vi "RDUW_2.0.vi"() -> ()   [LabVIEW 2010]
panel:
  in  "Reset":bool
  out "Previous Write time (sec)":dbl
  in  "Start writing":bool
  out "Rubbish variable":bool
  out "XY Graph":cluster{"Y":dbl[], "Y":dbl[]}[](graph)
  in  "Monitor Motor Position":bool=TRUE
  out "Program runtime (s)":dbl format="%.1f"
  in  "Go Origin":bool
  in  "Emergency STOP !!":bool caption="Emergency Button"
  out "Output Array":dbl[][](array[numeric])
  in  "Command":string
  out "Loop count":i32
  out "y":i32
  out "x":i32
  out "x-disp":i32[](array[numeric])
  out "y-disp":i32[](array[numeric])
  in  "Laser GPIB":u8=10
  in  "Motor GPIB":u8=6
  # "1) LINE<space>[Displacement]<space>[Speed]<space>[Current]<space>[t(on)]<space>[t(off)]"
  # "2) JUMP<space>[Displacement]<space>[Speed]"
  # "3) ARC<space>[Type]<space>[Radius]<space>[Current]<space>[t(on)]<space>[t(off)]"
  # "4) LINE1<space>[Displacement]<space>[Speed]<space>[Current]<space>[t_before]<space>[t_enable]<space>[Frequency]<space>[DTY]<space>[HIL]<space>[LOL]"
  # "5) LINE2<space>[Displacement]<space>[Speed]<space>[Current]<space>[t_before]<space>[frequency]<space>[Amplitude]<space>[t_enable]"
  # "6) WAIT<space>[time_ms]"
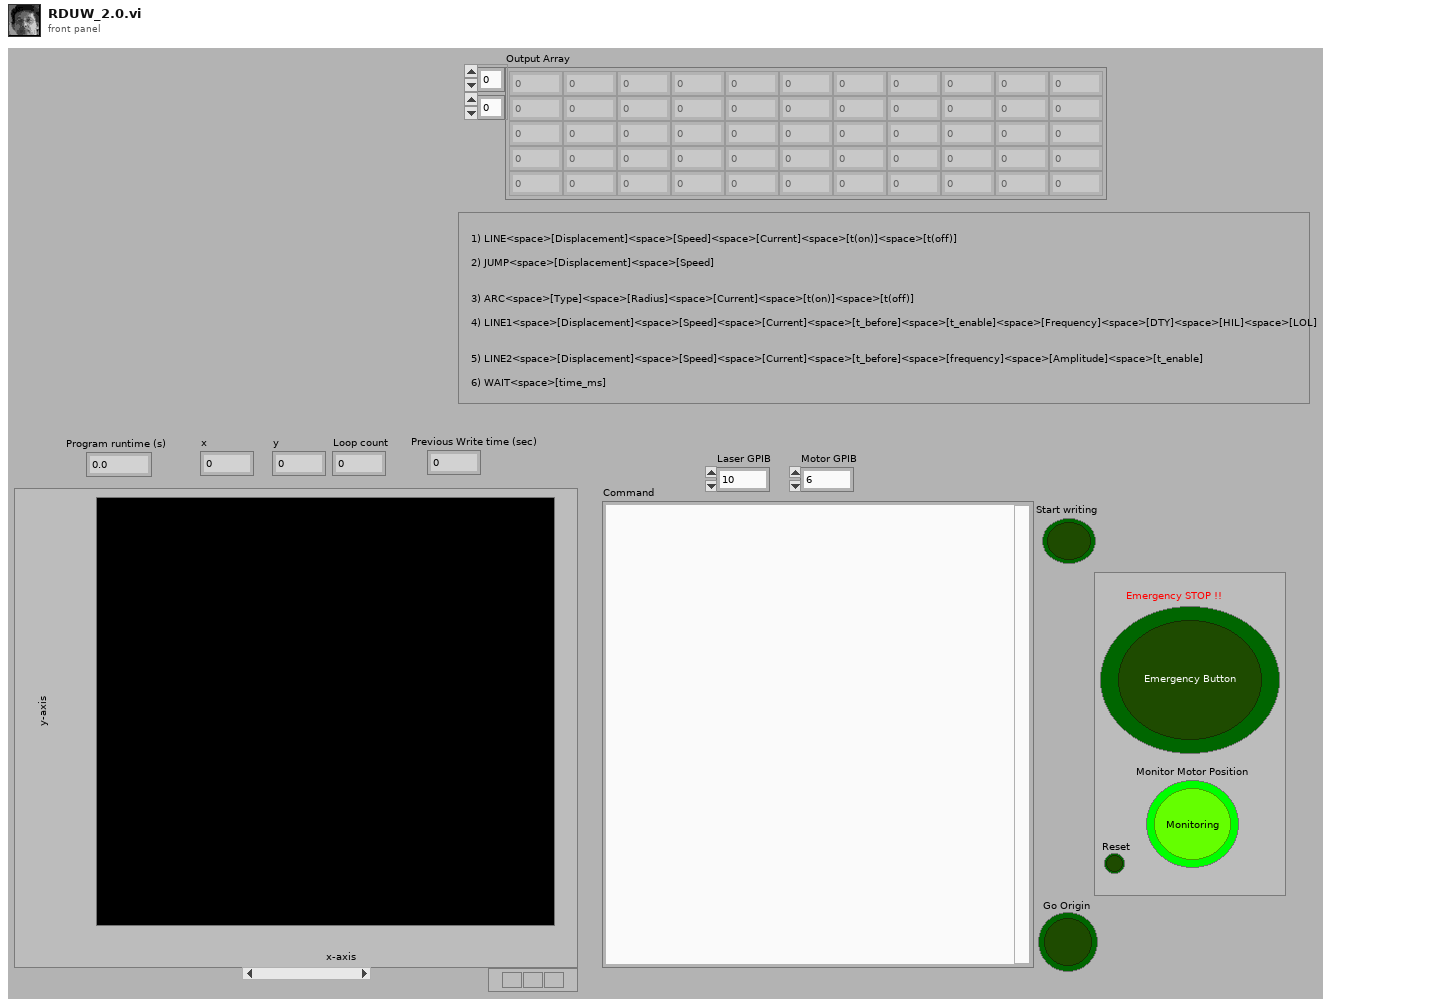
[diagram p1: front panel]
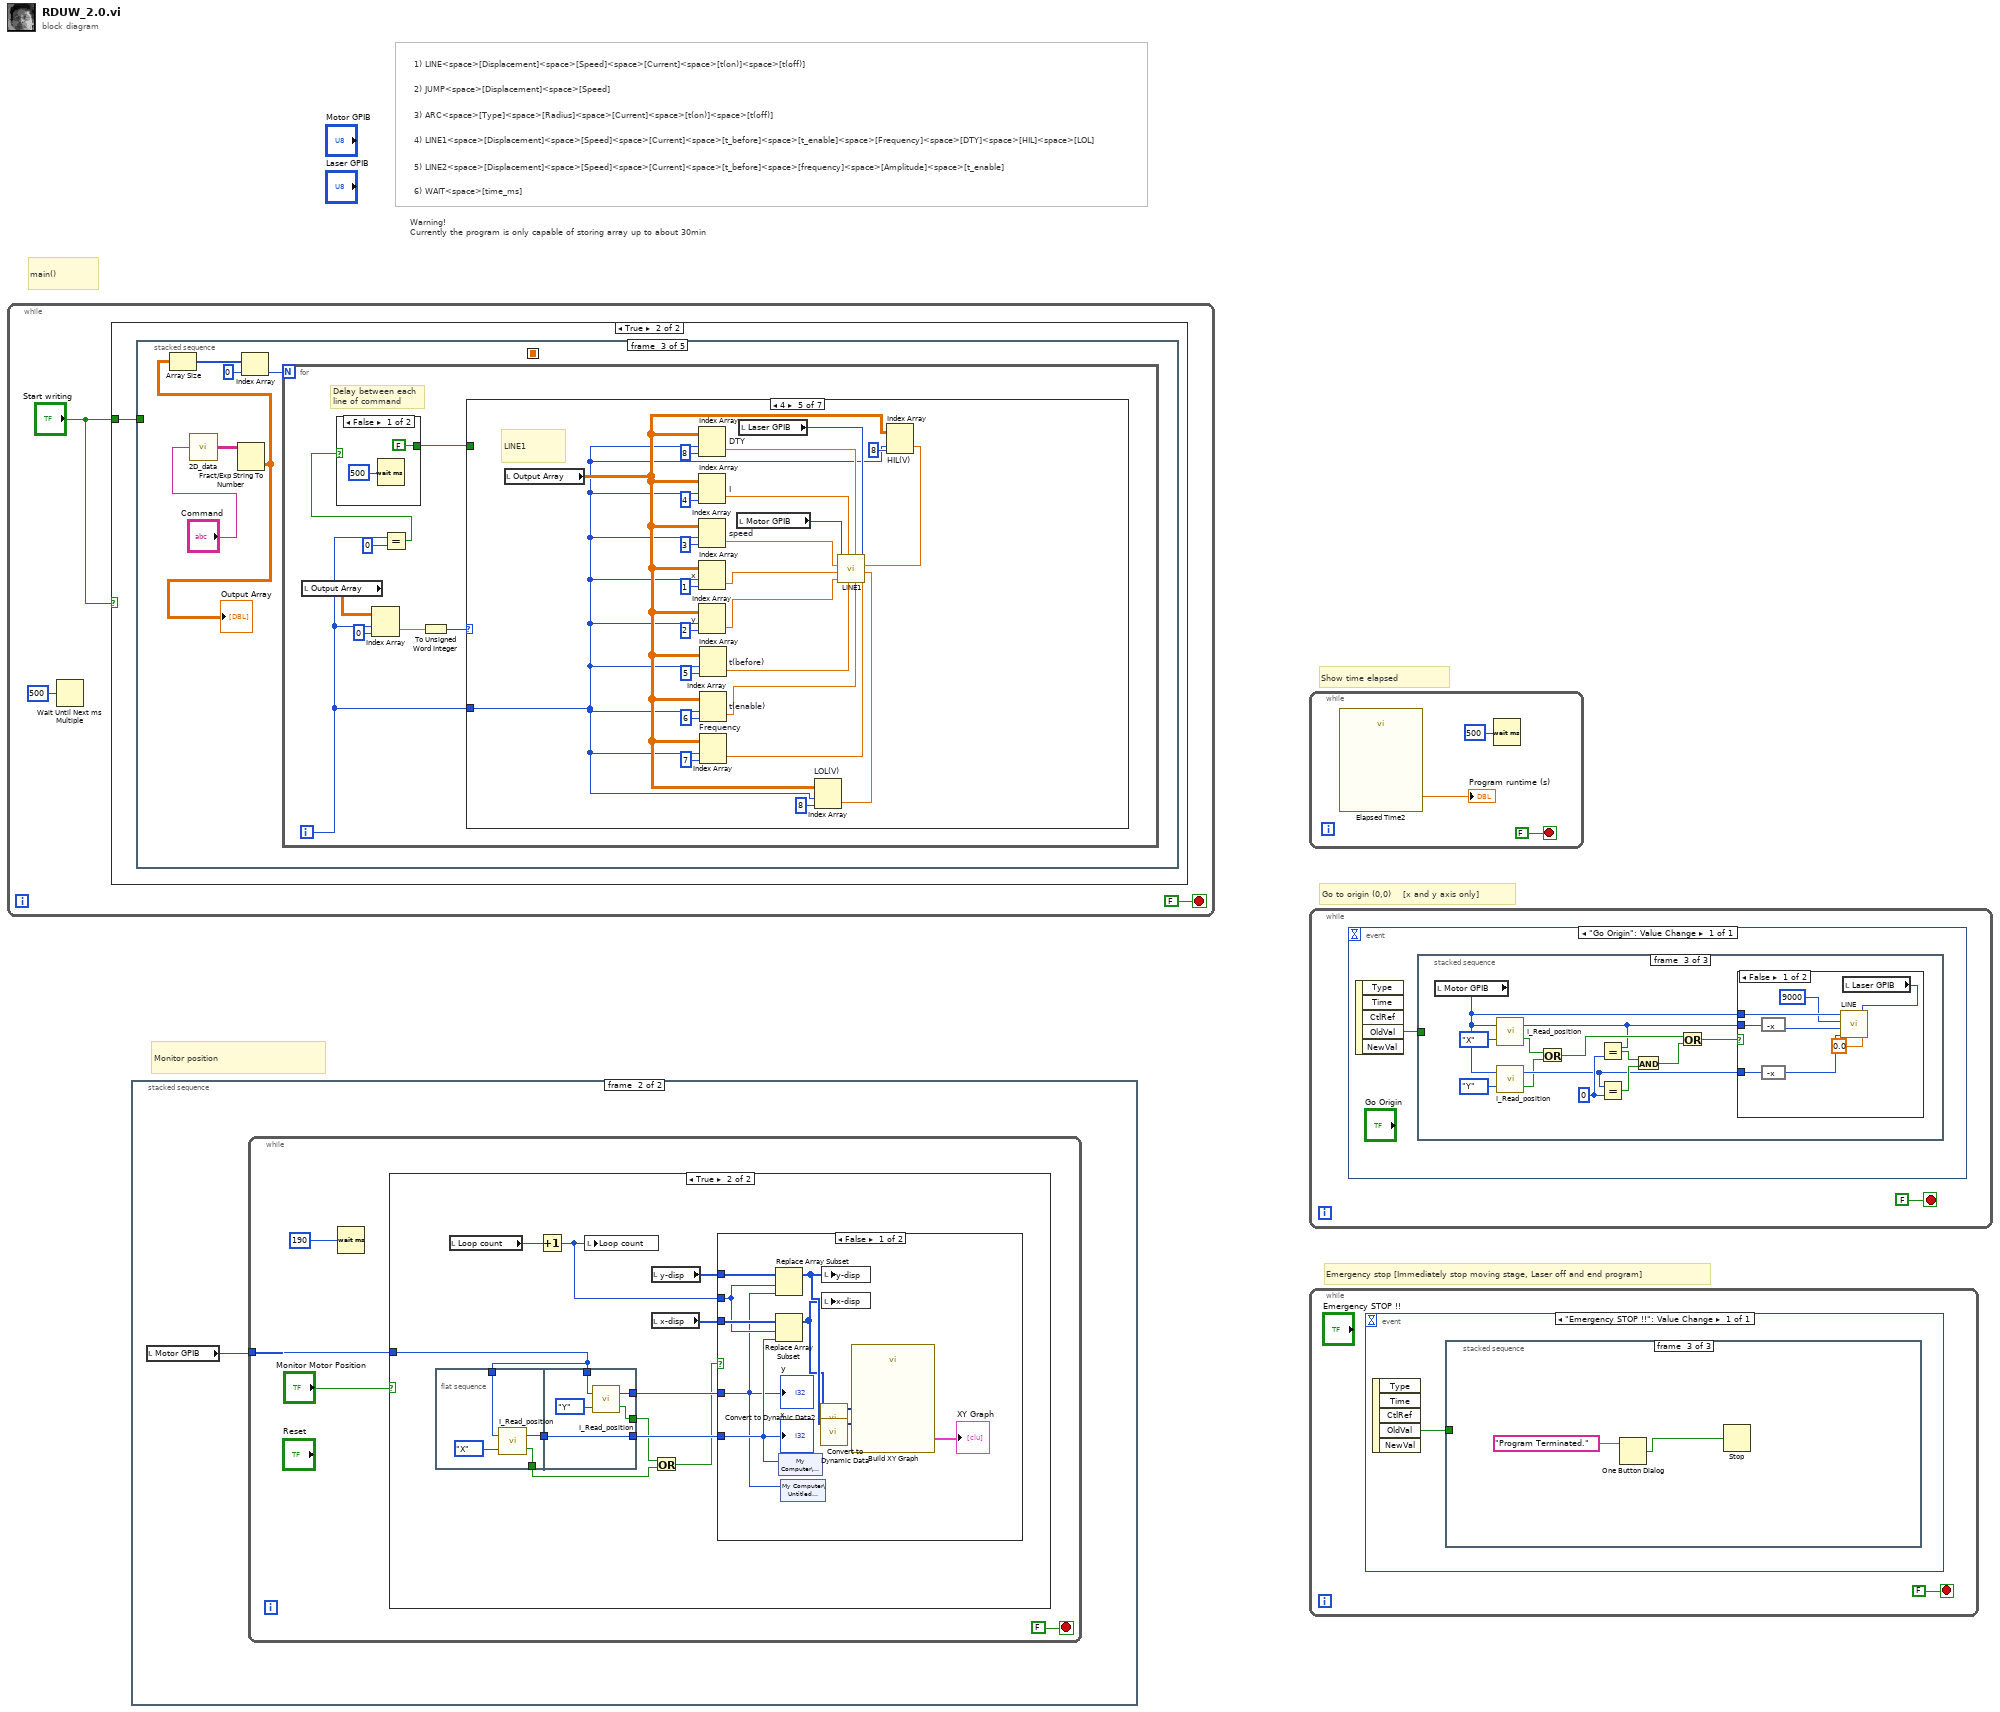
[diagram p0: block diagram]
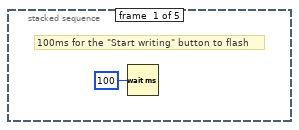
[diagram p3: hidden frame]
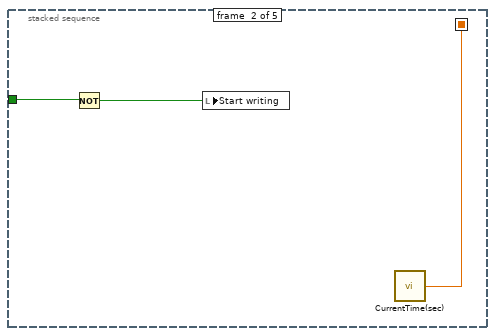
[diagram p4: hidden frame]
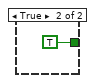
[diagram p5: hidden frame]
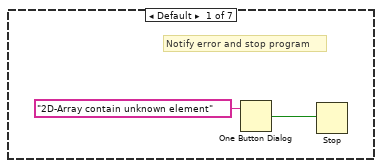
[diagram p6: hidden frame]
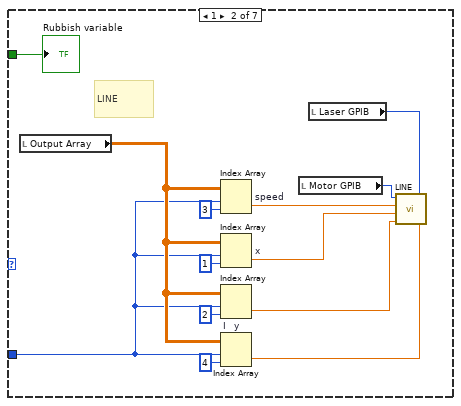
[diagram p7: hidden frame]
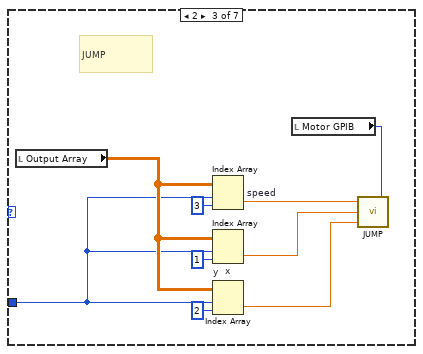
[diagram p8: hidden frame]
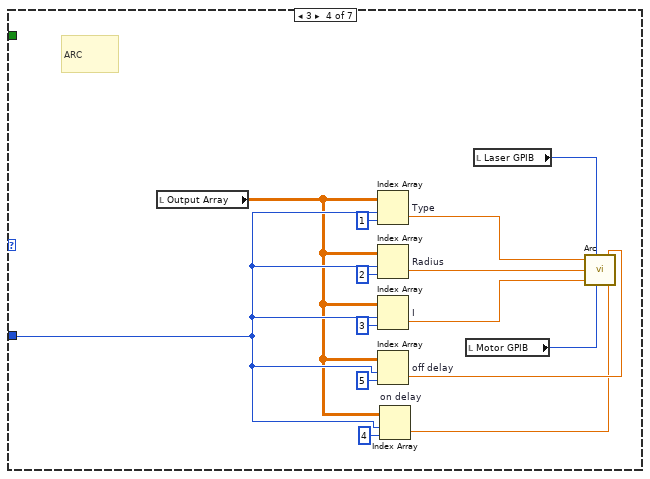
[diagram p9: hidden frame]
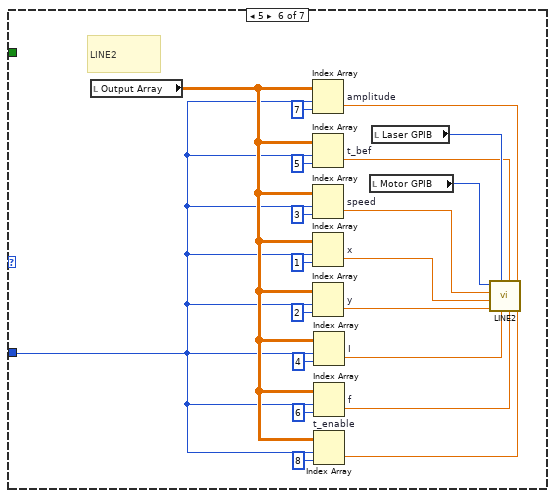
[diagram p10: hidden frame]
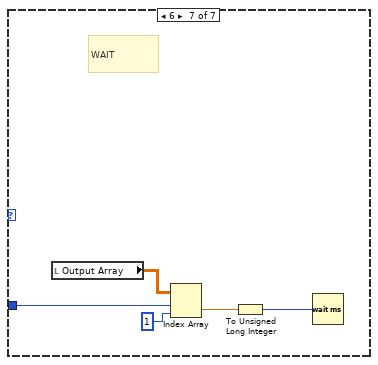
[diagram p11: hidden frame]
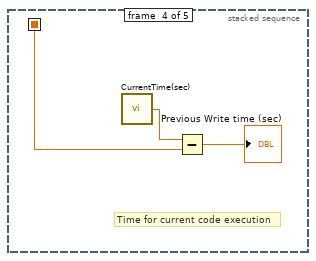
[diagram p12: hidden frame]
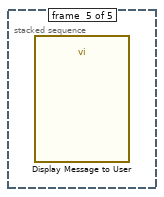
[diagram p13: hidden frame]
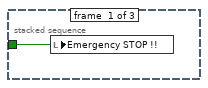
[diagram p14: hidden frame]
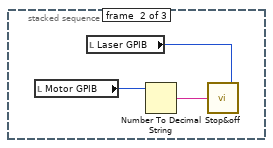
[diagram p15: hidden frame]
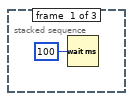
[diagram p16: hidden frame]
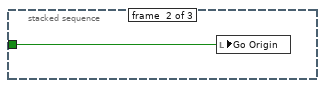
[diagram p17: hidden frame]
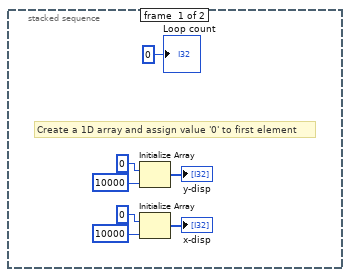
[diagram p19: hidden frame]
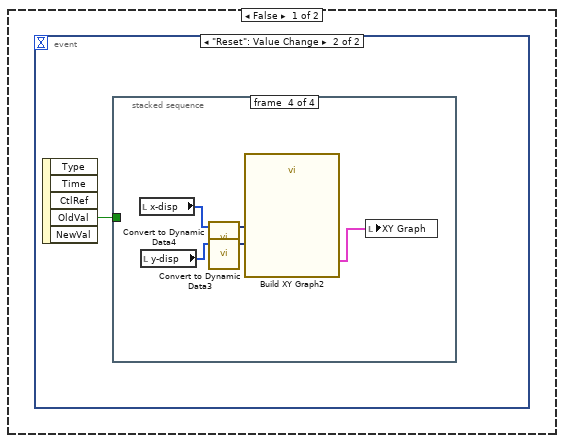
[diagram p20: hidden frame]
diagram:
  # "Warning!\nCurrently the program is only capable of storing array up to about 30min"
  # "main()"
  # "Emergency stop [Immediately stop moving stage, Laser off and end program]"
  # "Go to origin (0,0)    [x and y axis only]"
  # "Show time elapsed"
  # "6) WAIT<space>[time_ms]"
  # "5) LINE2<space>[Displacement]<space>[Speed]<space>[Current]<space>[t_before]<space>[frequency]<space>[Amplitude]<space>[t_enable]"
  # "Monitor position"
  # "4) LINE1<space>[Displacement]<space>[Speed]<space>[Current]<space>[t_before]<space>[t_enable]<space>[Frequency]<space>[DTY]<space>[HIL]<space>[LOL]"
  # "3) ARC<space>[Type]<space>[Radius]<space>[Current]<space>[t(on)]<space>[t(off)]"
  # "2) JUMP<space>[Displacement]<space>[Speed]"
  # "1) LINE<space>[Displacement]<space>[Speed]<space>[Current]<space>[t(on)]<space>[t(off)]"
  n1 = while {
    stop <- FALSE stop-if-true
    n2 = Wait Until Next ms Multiple(millisecond multiple=u32 500) -> ()  [unwired: 1 out]
    n3 = case shown="True" "Start writing" {
      tunnel: "Start writing" -> [_ w4]
      frame False {
      }
      frame True {
        n4 = stacked-sequence {
          seq-local: [_ w8 _ _ _] -> [_ _ _ w114 _]
          tunnel: w4 -> [_ w7 _ _ _]
          frame #0 {
            # "100ms for the \"Start writing\" button to flash"
            n5 = Wait (ms)(milliseconds to wait=u32 100) -> ()  [unwired: 1 out]
          }
          frame #1 {
            n6 = Not(x=w7) -> (.not. x?=w6:bool)
            n7 = local write "Start writing"(w6) -> ()
            n8 = call "CurrentTime(sec).vi"() -> ("CurrentTime(sec)"=w8:dbl)  [unwired: 1 in]
          }
          frame #2 {
            n9 = call "2D_data.vi"("String"="Command") -> ("output array"=w10:string[][])
            n10 = Fract/Exp String To Number(string=w10) -> (number=w9:dbl[][])  [unwired: 3 in, 1 out]
            "Output Array" <- w9
            n11 = Array Size(array=w9) -> (size(s)=w13:i32[])
            n12 = Index Array(array=w13, index=0) -> (element=w14:i32)
            n13 = for {
              N: w14 -> [_]
              i -> [w18]
              # "Delay between each\nline of command"
              n14 = local read "Output Array"() -> (w19:dbl[][])
              n15 = Index Array(array=w19, index (row)=w18, index (col)=0 ("disabled index (col)")) -> (element=w20:dbl)
              n16 = Equal?(x=w18, y=0) -> (x = y?=w16:bool)
              n17 = case shown="False" w16 {
                tunnel: [FALSE TRUE] -> w15
                frame False {
                  n18 = Wait (ms)(milliseconds to wait=u32 500) -> ()  [unwired: 1 out]
                }
                frame True {
                }
              }
              n19 = To Unsigned Word Integer(number=w20) -> (unsigned 16bit integer=w21:u16)
              n20 = case shown="4" w21 {
                tunnel: w18 -> [_ w28 w44 w63 w64 w88 w111]
                tunnel: w15 -> [_ w30 _ _ _ _ _]
                frame Default {
                  # "Notify error and stop program"
                  n21 = One Button Dialog(message="2D-Array contain unknown element") -> (true=w26:bool)  [unwired: 1 in]
                  n22 = Stop(stop? (T)=w26) -> ()
                }
                frame 1 {
                  # "LINE"
                  n23 = local read "Output Array"() -> (w29:dbl[][])
                  n24 = Index Array "speed"(array=w29, index (row)=w28, index (col)=3 ("disabled index (col)")) -> (element=w31:dbl)
                  n25 = Index Array "x"(array=w29, index (row)=w28, index (col)=1 ("disabled index (col)")) -> (element=w33:dbl)
                  n26 = Index Array "y"(array=w29, index (row)=w28, index (col)=2 ("disabled index (col)")) -> (element=w32:dbl)
                  n27 = Index Array "I"(array=w29, index (row)=w28, index (col)=4 ("disabled index (col)")) -> (element=w37:dbl)
                  n28 = local read "Motor GPIB"() -> (w39:u8)
                  n29 = local read "Laser GPIB"() -> (w40:u8)
                  n30 = call "LINE.vi"("Current (mA)"=w37, "Laser GPIB"=w40, "y-dist"=w32, "x-dist"=w33, "speed"=w31, "Motor GPIB"=w39) -> ()  [unwired: 2 in]
                  "Rubbish variable" <- w30
                }
                frame 2 {
                  # "JUMP"
                  n31 = local read "Output Array"() -> (w45:dbl[][])
                  n32 = Index Array "speed"(array=w45, index (row)=w44, index (col)=3 ("disabled index (col)")) -> (element=w43:dbl)
                  n33 = Index Array "x"(array=w45, index (row)=w44, index (col)=1 ("disabled index (col)")) -> (element=w42:dbl)
                  n34 = Index Array "y"(array=w45, index (row)=w44, index (col)=2 ("disabled index (col)")) -> (element=w41:dbl)
                  n35 = local read "Motor GPIB"() -> (w49:u8)
                  n36 = call "JUMP.vi"("Motor GPIB"=w49, "y-dist"=w41, "x-dist"=w42, "speed"=w43) -> ()
                }
                frame 3 {
                  # "ARC"
                  n37 = local read "Output Array"() -> (w52:dbl[][])
                  n38 = Index Array "Type"(array=w52, index (row)=w63, index (col)=1 ("disabled index (col)")) -> (element=w58:dbl)
                  n39 = Index Array "Radius"(array=w52, index (row)=w63, index (col)=2 ("disabled index (col)")) -> (element=w57:dbl)
                  n40 = Index Array "I"(array=w52, index (row)=w63, index (col)=3 ("disabled index (col)")) -> (element=w59:dbl)
                  n41 = Index Array "off delay"(array=w52, index (row)=w63, index (col)=5 ("disabled index (col)")) -> (element=w51:dbl)
                  n42 = Index Array "on delay"(array=w52, index (row)=w63, index (col)=4 ("disabled index (col)")) -> (element=w50:dbl)
                  n43 = local read "Motor GPIB"() -> (w55:u8)
                  n44 = local read "Laser GPIB"() -> (w56:u8)
                  n45 = call "Arc.vi"("Type"=w58, "Laser GPIB"=w56, "Radius"=w57, "Current (mA)"=w59, "Motor GPIB"=w55, "off delay"=w51, "on delay"=w50) -> ()
                }
                frame 4 {
                  # "LINE1"
                  n46 = local read "Output Array"() -> (w65:dbl[][])
                  n47 = Index Array "DTY"(array=w65, index (row)=w64, index (col)=8 ("disabled index (col)")) -> (element=w78:dbl)
                  n48 = Index Array "I"(array=w65, index (row)=w64, index (col)=4 ("disabled index (col)")) -> (element=w77:dbl)
                  n49 = Index Array "speed"(array=w65, index (row)=w64, index (col)=3 ("disabled index (col)")) -> (element=w76:dbl)
                  n50 = Index Array "x"(array=w65, index (row)=w64, index (col)=1 ("disabled index (col)")) -> (element=w75:dbl)
                  n51 = Index Array "y"(array=w65, index (row)=w64, index (col)=2 ("disabled index (col)")) -> (element=w74:dbl)
                  n52 = Index Array "t(before)"(array=w65, index (row)=w64, index (col)=5 ("disabled index (col)")) -> (element=w73:dbl)
                  n53 = Index Array "t(enable)"(array=w65, index (row)=w64, index (col)=6 ("disabled index (col)")) -> (element=w72:dbl)
                  n54 = Index Array "Frequency"(array=w65, index (row)=w64, index (col)=7 ("disabled index (col)")) -> (element=w71:dbl)
                  n55 = local read "Motor GPIB"() -> (w70:u8)
                  n56 = local read "Laser GPIB"() -> (w79:u8)
                  n57 = Index Array "LOL(V)"(array=w65, index (row)=w64, index (col)=8 ("disabled index (col)")) -> (element=w66:dbl)
                  n58 = Index Array "HIL(V)"(array=w65, index (row)=w64, index (col)=8 ("disabled index (col)")) -> (element=w67:dbl)
                  n59 = call "LINE1.vi"("Frequency(Hz)"=w71, "LOL(V)"=w66, "HIL(V)"=w67, "Laser GPIB"=w79, "Enable time(ms)"=w72, "DTY"=w78, "t_before(ms)"=w73, "Current (mA)"=w77, "y-dist"=w74, "x-dist"=w75, "speed"=w76, "Motor GPIB"=w70) -> ()
                }
                frame 5 {
                  # "LINE2"
                  n60 = local read "Output Array"() -> (w99:dbl[][])
                  n61 = Index Array "amplitude"(array=w99, index (row)=w88, index (col)=7 ("disabled index (col)")) -> (element=w90:dbl)
                  n62 = Index Array "t_bef"(array=w99, index (row)=w88, index (col)=5 ("disabled index (col)")) -> (element=w91:dbl)
                  n63 = Index Array "speed"(array=w99, index (row)=w88, index (col)=3 ("disabled index (col)")) -> (element=w95:dbl)
                  n64 = Index Array "x"(array=w99, index (row)=w88, index (col)=1 ("disabled index (col)")) -> (element=w96:dbl)
                  n65 = Index Array "y"(array=w99, index (row)=w88, index (col)=2 ("disabled index (col)")) -> (element=w94:dbl)
                  n66 = Index Array "I"(array=w99, index (row)=w88, index (col)=4 ("disabled index (col)")) -> (element=w93:dbl)
                  n67 = Index Array "f"(array=w99, index (row)=w88, index (col)=6 ("disabled index (col)")) -> (element=w92:dbl)
                  n68 = Index Array "t_enable"(array=w99, index (row)=w88, index (col)=8 ("disabled index (col)")) -> (element=w89:dbl)
                  n69 = local read "Motor GPIB"() -> (w98:u8)
                  n70 = local read "Laser GPIB"() -> (w97:u8)
                  n71 = call "LINE2.vi"("Enable time(ms)"=w89, "Amplitude(mV)"=w90, "Frequency(Hz)"=w92, "t_before(ms)"=w91, "Current (mA)"=w93, "Laser GPIB"=w97, "y-dist"=w94, "x-dist"=w96, "speed"=w95, "Motor GPIB"=w98) -> ()  [unwired: 2 in]
                }
                frame 6 {
                  # "WAIT"
                  n72 = local read "Output Array"() -> (w110:dbl[][])
                  n73 = Index Array "Index array"(array=w110, index (row)=w111, index (col)=1 ("disabled index (col)")) -> (element=w109:dbl)
                  n74 = To Unsigned Long Integer(number=w109) -> (unsigned 32bit integer=w108:u32)
                  n75 = Wait (ms)(milliseconds to wait=w108) -> ()  [unwired: 1 out]
                }
              }
            }
          }
          frame #3 {
            # "Time for current code execution"
            n76 = call "CurrentTime(sec).vi"() -> ("CurrentTime(sec)"=w115:dbl)  [unwired: 1 in]
            n77 = Subtract(x=w115, y=w114) -> (x-y=→"Previous Write time (sec)":dbl)
          }
          frame #4 {
            n78 = call "Display Message to User"() -> ()  [unwired: 10 in, 2 out]
          }
        }
      }
    }
  }
  n79 = stacked-sequence {
    frame #0 {
      # "Create a 1D array and assign value '0' to first element"
      n80 = Initialize Array(0 ("element"), 10000 ("dimension size")) -> (→"y-disp":i32[])
      n81 = Initialize Array(0 ("element"), 10000 ("element")) -> (→"x-disp":i32[])
      "Loop count" <- 0 ("Loop count")
    }
    frame #1 {
      n82 = local read "Motor GPIB"() -> (w123:u8)
      n83 = while {
        tunnel: w123 -> [w127]
        stop <- FALSE stop-if-true
        n84 = Wait (ms)(milliseconds to wait=u32 190 ("millisecond multiple")) -> ()  [unwired: 1 out]
        n85 = case shown="True" "Monitor Motor Position" {
          tunnel: w127 -> [_ w152]
          frame False {
            n86 = event shown="[1] \"Reset\": Value Change" {
              selector: _ -> [_ _]
              dyn-events: _ -> [_ _]
              timeout: _ -> [_ _]
              event "Monitor Motor Position": Value Change {
                n87 = event-data() -> ()  [unwired: 1 in, 5 out]
              }
              event "Reset": Value Change {
                n88 = event-data() -> ("OldVal"=w128:bool)  [unwired: 1 in, 4 out]
                n89 = stacked-sequence {
                  tunnel: w128 -> [_ w130 _ _]
                  frame #0 {
                    n90 = Wait (ms)(milliseconds to wait=u32 100) -> ()  [unwired: 1 out]
                  }
                  frame #1 {
                    n91 = local write "Reset"(w130) -> ()
                  }
                  frame #2 {
                    n92 = Initialize Array(0 ("element"), 10000 ("dimension size")) -> (w131:i32[])
                    n93 = Initialize Array(0 ("element"), 10000 ("element")) -> (w132:i32[])
                    n94 = local write "x-disp"(w131) -> ()
                    n95 = local write "y-disp"(w132) -> ()
                  }
                  frame #3 {
                    n96 = local read "x-disp"() -> (w138:i32[])
                    n97 = local read "y-disp"() -> (w137:i32[])
                    n98 = call "Convert to Dynamic Data4"("Array"=w138) -> ("Dynamic Data Type"=w140:dynamicdata)  [unwired: 3 in]
                    n99 = call "Convert to Dynamic Data3"("Array"=w137) -> ("Dynamic Data Type"=w141:dynamicdata)  [unwired: 3 in]
                    n100 = call "Build XY Graph2"("Y Input"=w141, "X Input"=w140) -> ("XY Graph"=w139:cluster{"Y":dbl[], "Y":dbl[]}[])  [unwired: 3 in, 6 out]
                    n101 = local write "XY Graph"(w139) -> ()
                  }
                }
              }
            }
          }
          frame True {
            n102 = flat-sequence {
              tunnel: w152 -> [w166]
              tunnel: [w164] -> w151
              tunnel: [w163] -> w145
              tunnel: w152 -> [w171]
              tunnel: [w170] -> w148
              tunnel: w151 -> [w168]
              tunnel: [w168] -> w147
              tunnel: [w167] -> w146
              frame #0 {
                n103 = call "I_Read_position.vi"("Axis"=enum16{"X", "Y", "Z"}."X", "Motor GPIB"=w166) -> ("Error?"=w163:bool, "Position"=w164:i32)
              }
              frame #1 {
                n104 = call "I_Read_position.vi"("Axis"=enum16{"X", "Y", "Z"}."Y", "Motor GPIB"=w171) -> ("Error?"=w167:bool, "Position"=w170:i32)
              }
            }
            n105 = local read "Loop count"() -> (w143:i32)
            n106 = Increment(x=w143) -> (x+1=w142:i32)
            n107 = local write "Loop count"(w142) -> ()
            n108 = local read "y-disp"() -> (w149:i32[])
            n109 = local read "x-disp"() -> (w150:i32[])
            n110 = Or(x=w146, y=w145) -> (x .or. y?=w144:bool)
            n111 = case shown="False" w144 {
              tunnel: w150 -> [w161 _]
              tunnel: w149 -> [w162 _]
              tunnel: w148 -> [w153 _]
              tunnel: w147 -> [w154 _]
              tunnel: w142 -> [w160 _]
              frame False {
                n112 = Replace Array Subset(array=w162, new element=w153, index=w160) -> (w158:i32[])
                n113 = Replace Array Subset(array=w161, new element=w154, index=w160) -> (w156:i32[])
                n114 = shared-variable "My Computer\\Untitled Library 3.lvlib\\x"(w154) -> ()  [unwired: 1 in, 1 out]
                n115 = shared-variable "My Computer\\Untitled Library 3.lvlib\\y"(w153) -> ()  [unwired: 1 in, 1 out]
                n116 = call "Convert to Dynamic Data2"("Array"=w156) -> ("Dynamic Data Type"=w155:dynamicdata)  [unwired: 3 in]
                n117 = call "Convert to Dynamic Data"("Array"=w158) -> ("Dynamic Data Type"=w157:dynamicdata)  [unwired: 3 in]
                n118 = local write "y-disp"(w158) -> ()
                n119 = local write "x-disp"(w156) -> ()
                n120 = call "Build XY Graph"("Y Input"=w157, "X Input"=w155) -> ("XY Graph"=→"XY Graph":cluster{"Y":dbl[], "Y":dbl[]}[])  [unwired: 3 in, 6 out]
                "y" <- w153
                "x" <- w154
              }
              frame True {
              }
            }
          }
        }
      }
    }
  }
  n121 = while {
    stop <- FALSE stop-if-true
    n122 = call "Elapsed Time2"() -> ("Elapsed Time (s)"=→"Program runtime (s)":dbl)  [unwired: 12 in, 7 out]
    n123 = Wait (ms)(milliseconds to wait=u32 500) -> ()  [unwired: 1 out]
  }
  n124 = while {
    stop <- FALSE stop-if-true
    n125 = event shown="[0] \"Go Origin\": Value Change" {
      selector: _ -> [_]
      dyn-events: _ -> [_]
      timeout: _ -> [_]
      event "Go Origin": Value Change {
        n126 = event-data() -> ("OldVal"=w176:bool)  [unwired: 1 in, 4 out]
        n127 = stacked-sequence {
          tunnel: w176 -> [_ w178 _]
          frame #0 {
            n128 = Wait (ms)(milliseconds to wait=u32 100) -> ()  [unwired: 1 out]
          }
          frame #1 {
            n129 = local write "Go Origin"(w178) -> ()
          }
          frame #2 {
            w186 = 0 ("y")
            n130 = local read "Motor GPIB"() -> (w181:u8)
            n131 = call "I_Read_position.vi"("Axis"=enum16{"X", "Y", "Z", "U"}."X", "Motor GPIB"=w181) -> ("Error?"=w182:bool, "Position"=w184:i32)
            n132 = call "I_Read_position.vi"("Axis"=enum16{"X", "Y", "Z", "U"}."Y", "Motor GPIB"=w181) -> ("Error?"=w183:bool, "Position"=w185:i32)
            n133 = Or(x=w182, y=w183) -> (x .or. y?=w190:bool)
            n134 = Equal?(x=w184, y=w186) -> (x = y?=w188:bool)
            n135 = Equal?(x=w185, y=w186) -> (x = y?=w187:bool)
            n136 = And(x=w188, y=w187) -> (x .and. y?=w189:bool)
            n137 = Or(x=w190, y=w189) -> (x .or. y?=w191:bool)
            n138 = case shown="False" w191 {
              tunnel: w181 -> [w199 _]
              tunnel: w184 -> [w197 _]
              tunnel: w185 -> [w196 _]
              frame False {
                n139 = expression code="-x"(w197) -> (w194:i32)
                n140 = expression code="-x"(w196) -> (w195:i32)
                n141 = local read "Laser GPIB"() -> (w192:u8)
                n142 = call "LINE.vi"("Current (mA)"=0.0, "Laser GPIB"=w192, "y-dist"=w195, "x-dist"=w194, "speed"=u16 9000, "Motor GPIB"=w199) -> ()  [unwired: 2 in]
              }
              frame True {
              }
            }
          }
        }
      }
    }
  }
  n143 = while {
    stop <- FALSE stop-if-true
    n144 = event shown="[0] \"Emergency STOP !!\": Value Change" {
      selector: _ -> [_]
      dyn-events: _ -> [_]
      timeout: _ -> [_]
      event "Emergency STOP !!": Value Change {
        n145 = event-data() -> ("OldVal"=w201:bool)  [unwired: 1 in, 4 out]
        n146 = stacked-sequence {
          tunnel: w201 -> [w202 _ _]
          frame #0 {
            n147 = local write "Emergency STOP !!"(w202) -> ()
          }
          frame #1 {
            n148 = local read "Motor GPIB"() -> (w204:u8)
            n149 = local read "Laser GPIB"() -> (w205:u8)
            n150 = Number To Decimal String(number=w204) -> (decimal integer string=w203:string)  [unwired: 1 in]
            n151 = call "Stop&off.vi"("Laser GPIB"=w205, "Motor GPIB"=w203) -> ()
          }
          frame #2 {
            n152 = One Button Dialog(message="Program Terminated.") -> (true=w206:bool)  [unwired: 1 in]
            n153 = Stop(stop? (T)=w206) -> ()
          }
        }
      }
    }
  }
